vi "Update Waveforms.vi"(8 "error in (no error)":errorcluster, 11 "Model in":refnum<class "Model.lvclass">) -> (0 "error out":errorcluster, 3 "Model out":refnum<class "Model.lvclass">)   [LabVIEW 2015, in "Model.lvclass"]
uses:
  Model.lvclass
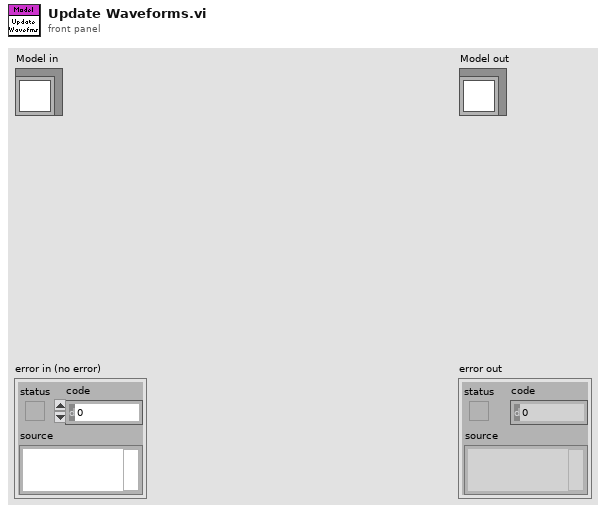
[diagram p1: front panel]
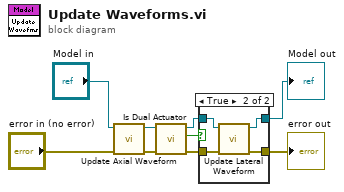
[diagram p0: block diagram]
diagram:
  n1 = call "Update Axial Waveform.vi"("error in (no error)"="error in (no error)", "Model in"="Model in") -> ("error out"=w5:errorcluster, "Model out"=w1:refnum<class "Model.lvclass">)  [unwired: 8 in]
  n2 = call "Is Dual Actuator.vi"("error in (no error)"=w5, "Model in"=w1) -> ("error out"=w4:errorcluster, "Is Dual Actuator"=w2:bool, "Model out"=w3:refnum<class "Model.lvclass">)  [unwired: 7 in]
  n3 = case shown="True" w2 {
    tunnel: w4 -> [w10 w15]
    tunnel: [w10 w14] -> w8
    tunnel: [w11 w13] -> w7
    tunnel: w3 -> [w11 w12]
    frame False {
    }
    frame True {
      n4 = call "Update Lateral Waveform.vi"("error in (no error)"=w15, "Model in"=w12) -> ("error out"=w14:errorcluster, "Model out"=w13:refnum<class "Model.lvclass">)  [unwired: 8 in]
    }
  }
  "error out" <- w8
  "Model out" <- w7
